vi "Test.vi"() -> ()   [LabVIEW 2012]
uses:
  <instrlib>/Ocean Server OS4000/Ocean Server OS4000.lvlib
panel:
  out "Angles 2":dbl[][](graph)
  in  "Heading PID Gains":T1={"proportional gain (Kc)"=1.0, "integral time (Ti, min)"=0.01, "derivative time (Td, min)"=0.0}
  in  "Heading Setpoint":dbl
  out "Pwm Output 2":dbl
  out "Pwm Output":dbl
  in  "Depth Setpoint":dbl
  in  "Depth PID Gains":T1={"proportional gain (Kc)"=1.0, "integral time (Ti, min)"=0.01, "derivative time (Td, min)"=0.0}
  in  "Baud Rate":u32(ring)=19200
  in  "Reset (True)":bool=TRUE
  in  "ID Query (False)":bool
  in  "VISA resource name":refnum<visa-resource-name>
  out "PSI":dbl(knob)
  in  "stop":bool
  in  "milliseconds to wait":u32=10
  in  "Atm Offset":dbl
  out "Actual Depth (m)":dbl(slide)
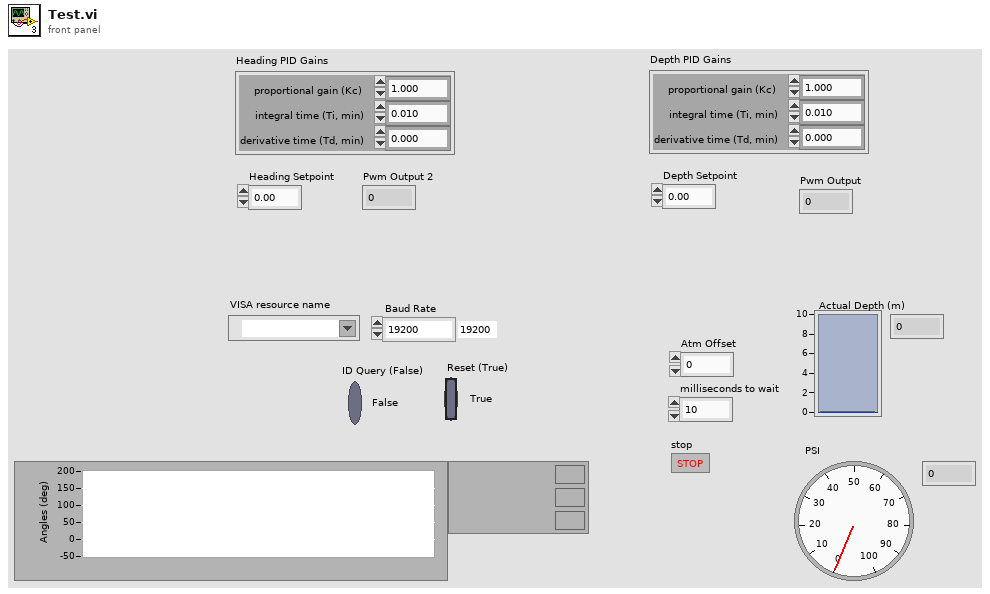
[diagram p1: front panel]
types:
  T1 = cluster{"proportional gain (Kc)":dbl, "integral time (Ti, min)":dbl, "derivative time (Td, min)":dbl}
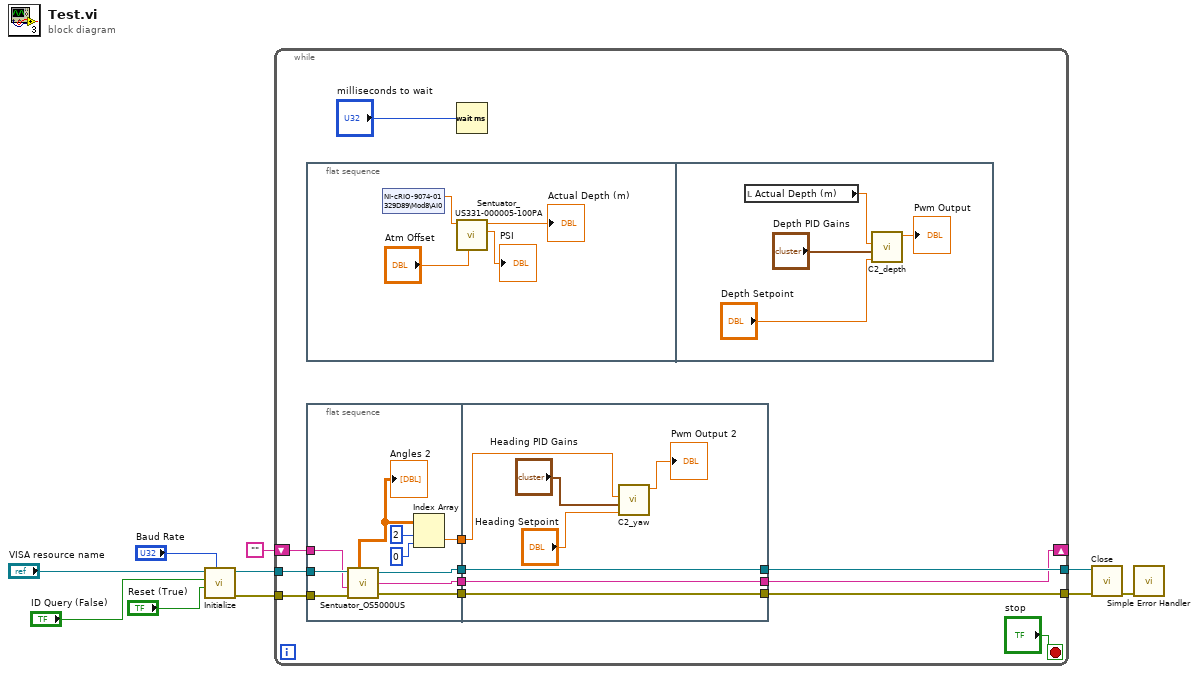
[diagram p0: block diagram]
diagram:
  n1 = call <instrlib>:"Initialize.vi"("Baud Rate"="Baud Rate", "Reset (True)"="Reset (True)", "ID Query (False)"="ID Query (False)", "VISA resource name"="VISA resource name") -> ("error out"=w5:errorcluster, "VISA resource name out"=w6:refnum<visa-resource-name>)  [unwired: 6 in]
  n2 = while {
    tunnel: w6 -> [w20]
    tunnel: w5 -> [w18]
    shift-right: [w12] -> _
    shift-left: "" -> [w19]
    tunnel: [w13] -> w2
    tunnel: [w11] -> w1
    stop <- "stop" stop-if-true
    n3 = flat-sequence {
      frame #0 {
        n4 = shared-variable "NI-cRIO-9074-01329D89\\Mod8\\AI0"() -> (w42:dbl)  [unwired: 1 in, 1 out]
        n5 = call "Sentuator_US331-000005-100PA.vi"("Atm Offset"="Atm Offset", "Depth sensor \nVoltage"=w42) -> ("PSI"=→"PSI":dbl, "Actual Depth (m)"=→"Actual Depth (m)":dbl)  [unwired: 7 in, 1 out]
      }
      frame #1 {
        n6 = local read "Actual Depth (m)"() -> (w45:dbl)
        n7 = call "C2_depth.vi"("setpoint"="Depth Setpoint", "PID gains"="Depth PID Gains", "Actual Depth"=w45) -> ("Pwm Output"=→"Pwm Output":dbl)
      }
    }
    n8 = flat-sequence {
      tunnel: w20 -> [w32]
      tunnel: w19 -> [w31]
      tunnel: w18 -> [w30]
      tunnel: [w29] -> w17
      tunnel: [w28] -> w16
      tunnel: [w27] -> w15
      tunnel: [w24] -> w14
      tunnel: w17 -> [w39]
      tunnel: w16 -> [w38]
      tunnel: w15 -> [w37]
      tunnel: w14 -> [w34]
      tunnel: [w39] -> w13
      tunnel: [w38] -> w12
      tunnel: [w37] -> w11
      frame #0 {
        n9 = call "Sentuator_OS5000US.vi"("VISA resource name"=w32, "Text to prepend to sentence"=w31, "error in (no error)"=w30) -> ("Angles"=w26:dbl[][], "VISA resource name out"=w29:refnum<visa-resource-name>, "Remaining Sentence"=w28:string, "error out"=w27:errorcluster)  [unwired: 1 in]
        "Angles 2" <- w26
        n10 = Index Array(array=w26, index (row)=2, index (col)=0) -> (element=w24:dbl)
      }
      frame #1 {
        n11 = call "C2_yaw.vi"("setpoint"="Heading Setpoint", "PID gains"="Heading PID Gains", "Actual Heading"=w34) -> ("Pwm Output"=→"Pwm Output 2":dbl)
      }
    }
    n12 = Wait (ms)(milliseconds to wait="milliseconds to wait") -> ()  [unwired: 1 out]
  }
  n13 = call <instrlib>:"Close.vi"("error in (no error)"=w1, "VISA resource name"=w2) -> ("error out"=w3:errorcluster)  [unwired: 9 in]
  n14 = call <vilib>:"Simple Error Handler.vi"("error in (no error)"=w3) -> ()  [unwired: 1 in, 8 out]
